vi "Calculate Data Rate.vi"(0 "device session in":refnum<class "Device Session.lvclass">, 5 "total samples fetched":u64, 11 "error in":errorcluster) -> (4 "device session out":refnum<class "Device Session.lvclass">, 6 "transfer rate (MB/s)":dbl, 15 "error out":errorcluster)   [LabVIEW 2015, in "Device Session.lvclass"]
doc: "Calculates the rate at which data is being acquired.\n\n<B>Input Parameters</B>\n\n<B>device session in</B> is a reference to the session containing sessions to all instrument design libraries used in this sample project. This parameter is obtained from the 'Open Session' VI.\n\n<B>total samples fetched</B> specifies the total number of samples fetched per channel since initiating acquisition.\n\n<B>error in</B> describes error conditions that occur before this node runs. This input provides standard 'error in' functionality.\n\n<B>Output Parameters</B>\n\n<B>device session out</B> passes a reference to the session to the next VI.\n\n<B>transfer rate (MB/s)</B> returns the average rate of acquisition.\n\n<B>error out</B> contains error information. This output provides standard 'error out' functionality."
uses:
  Device Session.lvclass
  Device Session.lvclass/Device Session.ctl
  <vilib>/Utility/error.llb/Error Cluster From Error Code.vi
  <vilib>/rvi/errors/niLvFpgaAdjustHostInterfaceError.vi
  <vilib>/rvi/interface/nirviReadWriteControl/nirviReadWriteControl.xnode
  FPGA Refnum.ctl
  NiFpgaLv.dll
  <vilib>/rvi/interface/Simulation/niFpgaSimulationCallBeginRW.vi
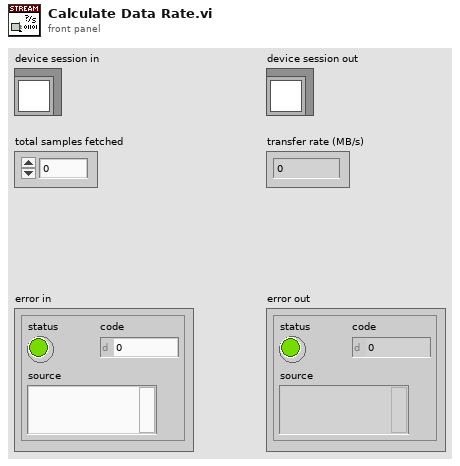
[diagram p1: front panel]
types:
  T1 = typedef "Device Session.lvclass/Device Session Object.ctl" = cluster{"ni5171R FPGA Reference":T2, "niHSAI config":refnum<class "niHSAI Config v1 Host.lvclass">, "configured scaling coefficients":cluster{"gain":dbl, "offset":dbl}[], "number of channels to stream":u8, "selected acq channels":bool[], "number of channels":u32, "actual channel configuration":T3[], "configured channels":bool[], "sample clock rate (Hz)":dbl}
  T2 = typedef "Device Session.lvclass/FPGA Refnum.ctl" = refnum<k20>
  T3 = typedef "niHSAI Types v1 Host.lvlib/Channel Configuration.ctl" = cluster{"channel":u32, "coupling":T4, "impedance":T5, "bandwidth":T6, "vertical range":dbl, "vertical offset":dbl}
  T4 = typedef "niHSAI Types v1 Host.lvlib/Coupling.ctl" = enum8{"Default", "DC", "AC"}
  T5 = typedef "niHSAI Types v1 Host.lvlib/Impedance.ctl" = enum8{"Default", "1 mega ohm", "50 ohm"}
  T6 = typedef "niHSAI Types v1 Host.lvlib/Bandwidth.ctl" = enum8{"Default", "Full Bandwidth", "Anti-alias Filter"}
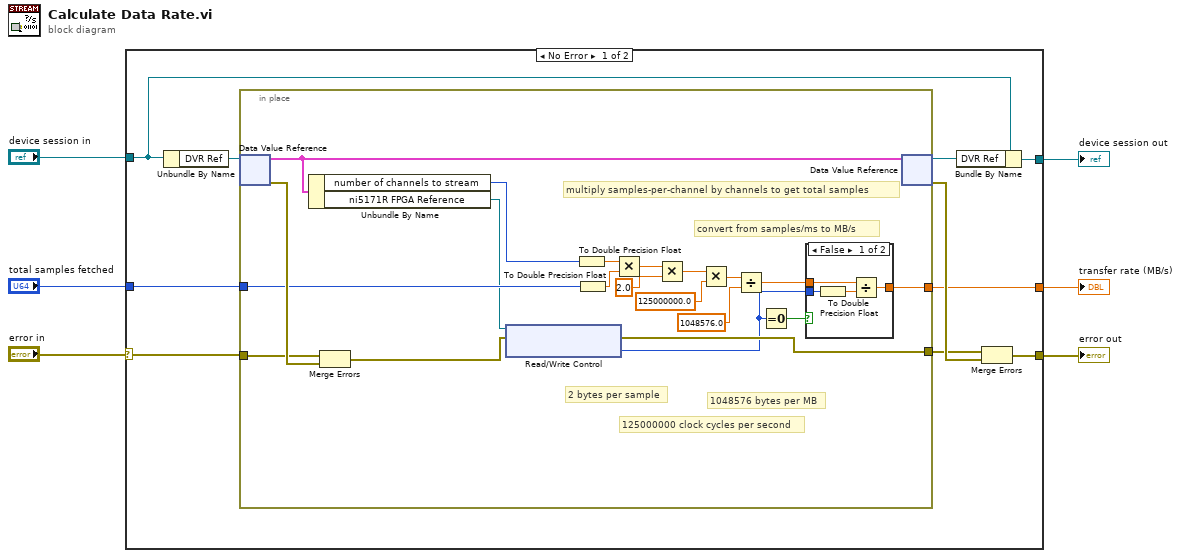
[diagram p0: block diagram]
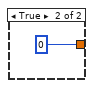
[diagram p2: hidden frame]
diagram:
  n1 = case shown="No Error" "error in" {
    selector: "error in" -> [w16 w43]
    tunnel: [w10 w42] -> w3
    tunnel: [w14 w43] -> w4
    tunnel: "device session in" -> [w9 w42]
    tunnel: [w8 _] -> w2
    tunnel: "total samples fetched" -> [w7 _]
    frame No Error {
      n2 = Unbundle By Name(w9) -> ("DVR Ref"=w12:refnum<data-value>)
      n3 = in-place {
        in-place-border: w16 -> [w35]
        in-place-border: [w18] -> w11
        in-place-border: [w26] -> w8
        in-place-border: w7 -> [w23]
        # "multiply samples-per-channel by channels to get total samples"
        # "2 bytes per sample"
        # "1048576 bytes per MB"
        # "125000000 clock cycles per second"
        # "convert from samples/ms to MB/s"
        n4 = in-place-dvr #1(w12) -> (w34:T1, w36:errorcluster)
        n5 = Unbundle By Name(w34) -> ("number of channels to stream"=w22:u8, "ni5171R FPGA Reference"=w19:T2)
        n6 = Merge Errors(w35, w36) -> (w20:errorcluster)
        n7 = xnode "Read/Write Control"("FPGA VI Reference In"=w19, "error in"=w20) -> ("error out"=w18:errorcluster, "status.clock cycles"=w17:u64)  [unwired: 1 out]
        n8 = To Double Precision Float(number=w22) -> (double precision float=w25:dbl)
        n9 = To Double Precision Float(number=w23) -> (double precision float=w21:dbl)
        n10 = Multiply(x=w25, y=w21) -> (x*y=w24:dbl)
        n11 = Multiply(x=w24, y=2.0) -> (x*y=w32:dbl)
        n12 = Multiply(x=w32, y=125000000.0) -> (x*y=w29:dbl)
        n13 = Divide(x=w29, y=1048576.0) -> (x/y=w31:dbl)
        n14 = Equal To 0?(x=w17) -> (x = 0?=w28:bool)
        n15 = case shown="False" w28 {
          tunnel: [w40 u64 0] -> w26
          tunnel: w31 -> [w38 _]
          tunnel: w17 -> [w37 _]
          frame False {
            n16 = To Double Precision Float(number=w37) -> (double precision float=w39:dbl)
            n17 = Divide(x=w38, y=w39) -> (x/y=w40:dbl)
          }
          frame True {
          }
        }
        n18 = in-place-dvr #1(w34) -> (w15:refnum<data-value>, w13:errorcluster)
      }
      n19 = Bundle By Name(cluster=w9, "DVR Ref"=w15) -> (w10:refnum<class "Device Session.lvclass">)
      n20 = Merge Errors(w11, w13) -> (w14:errorcluster)
    }
    frame Error {
    }
  }
  "transfer rate (MB/s)" <- w2
  "device session out" <- w3
  "error out" <- w4
